vi "Write Witness.vi"(8 "error in":errorcluster, 10 "Witness":string, 11 "Base Software in":refnum<class "Main.lvclass">) -> (0 "error out":errorcluster, 3 "Base Software out":refnum<class "Main.lvclass">)   [LabVIEW 2023, in "Main.lvlib" / "Main.lvclass"]
uses:
  Project/Main.lvclass
  Project/Main.lvclass/Main.ctl
  Custom Controls/Color_Items.ctl
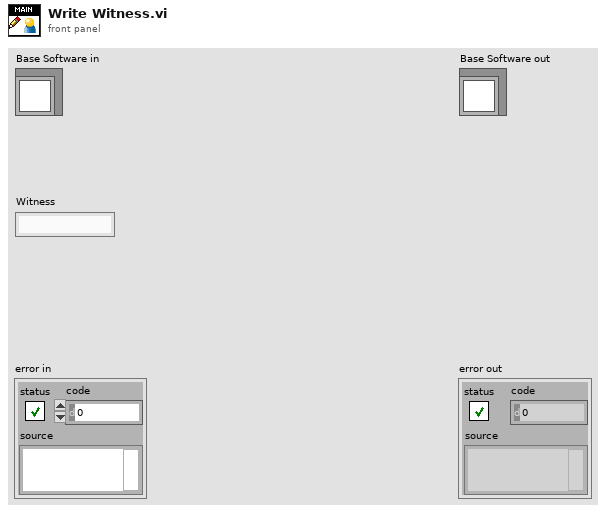
[diagram p1: front panel]
types:
  T1 = typedef "Main.lvlib/Main.lvclass/Color_Items.ctl" = enum16{"Nominal_Low_Impact", "Nominal", "User_Interaction", "Warning", "Error"}
  T2 = typedef "LVTextColorsTypeDef.ctl" = cluster{"Text Color":u32, "Background Color":u32}
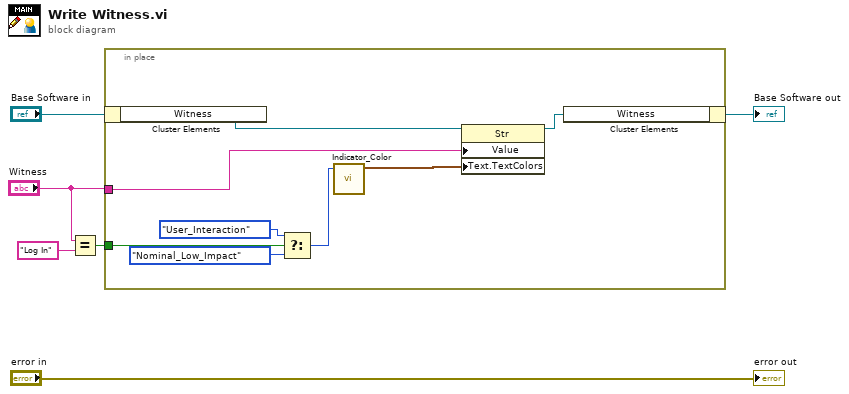
[diagram p0: block diagram]
diagram:
  n1 = Equal?(x="Witness", y="Log In") -> (x = y?=w2:bool)
  n2 = in-place {
    in-place-border: "Witness" -> [w13]
    in-place-border: w2 -> [w11]
    n3 = in-place-cluster #1("Base Software in") -> ("Witness"=w8:refnum<vi>)
    n4 = Select(t=Color_Items."User_Interaction" ("Color Selector"), s=w11, f=Color_Items."Nominal_Low_Impact" ("Color Selector")) -> (s? t:f=w9:T1)
    n5 = call "Indicator_Color.vi"("Color Selector"=w9) -> ("Text Colors"=w14:T2)  [unwired: 10 in]
    n6 = property class="Str"(reference=w8, "Value"=w13, "Text.TextColors"=w14) -> (reference out=w7:refnum<vi>)  [unwired: 1 in, 1 out]
    n7 = in-place-cluster #1("Witness"=w7) -> (→"Base Software out":refnum<class "Main.lvclass">)
  }
  "error out" <- "error in"
